vi "Nested CLI and File.vi"   [LabVIEW 2020, in "Caraya Extension Tests.lvclass"]
uses:
  Caraya Extension Tests.lvclass
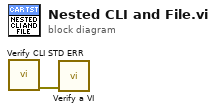
[diagram p0: block diagram]
diagram:
  n1 = call "Verify CLI STD ERR.vi"() -> ("error out"=w1:errorcluster)  [unwired: 11 in]
  n2 = call "Verify a VI.vi"("error in"=w1) -> ()  [unwired: 10 in, 1 out]
